vi "CombiningVIs.vi"() -> ()   [LabVIEW 2012]
uses:
  SubVIs/LVPresent_Globals.vi
  BotSpeakSubs/BotspeakSettingsUsed.vi
panel:
  in  "State 2":enum16{"LO", "HI"}(ring)=enum."HI"
  in  "Open":bool
  in  "Port":u8=13
  in  "State":enum16{"LO", "HI"}(ring)
  in  "Run":bool
  # "Combining VIs\n\nYou can add multiple VIs together on the diagram - and if you wire them together, the pink line defines the order in which things execute.  Wires contain data, and the second VI on a string cannot run until the first is complete and puts data on the pink wire.  If there were no wire, both VIs would run at the same time.  First click the Run button again, and then try opening the VI and playing around with the code."
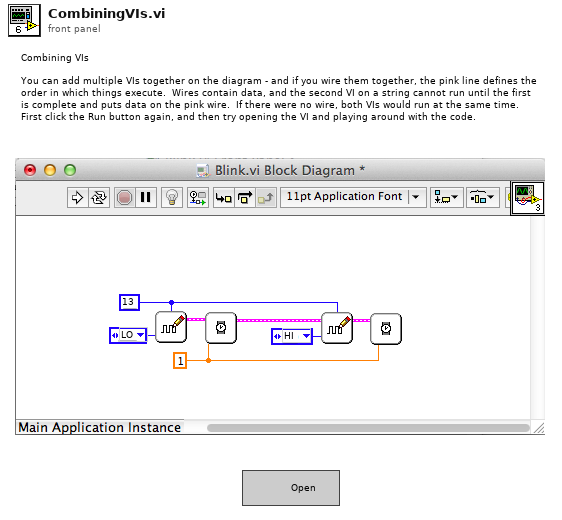
[diagram p1: front panel]
types:
  T1 = typedef "BotSpeak_Control.ctl" = cluster{"Address":string, "Reply EOF":string, "Hardware":string, "Retries":i8, "Timeout":i32, "Open?":bool}
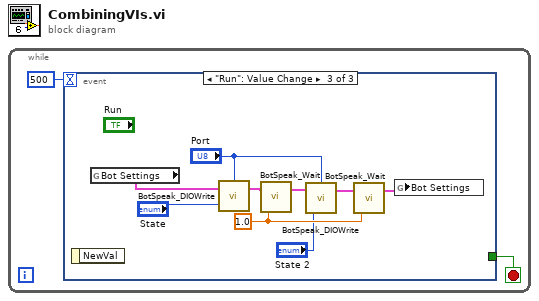
[diagram p0: block diagram]
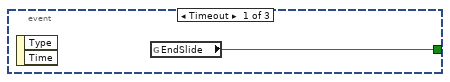
[diagram p2: hidden frame]
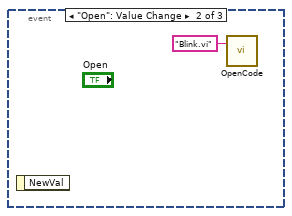
[diagram p3: hidden frame]
diagram:
  n1 = while {
    stop <- w2 stop-if-true
    n2 = event shown="[2] \"Run\": Value Change" {
      selector: _ -> [_ _ _]
      dyn-events: _ -> [_ _ _]
      timeout: 500 -> [_ _ _]
      tunnel: [w3 _ _] -> w2
      event Timeout {
        n3 = event-data() -> ()  [unwired: 1 in, 2 out]
        n4 = global read "LVPresent_Globals.vi" "EndSlide"() -> (w3:bool)
      }
      event "Open": Value Change {
        n5 = event-data() -> ()  [unwired: 1 in, 1 out]
        n6 = call "OpenCode.vi"("Code name"="Blink.vi") -> ()  [unwired: 3 in]
      }
      event "Run": Value Change {
        w9 = 1.0 ("Wait (sec)")
        n7 = event-data() -> ()  [unwired: 1 in, 1 out]
        n8 = global read "BotspeakSettingsUsed.vi" "Bot Settings"() -> (w6:T1)
        n9 = call <userlib>:"BotSpeak_DIOWrite.vi"("State"="State", "Bot Settings"=w6, "DIO Line"="Port") -> ("Bot Settings"=w12:T1)  [unwired: 1 out]
        n10 = call <userlib>:"BotSpeak_Wait.vi"("Wait (sec)"=w9, "Bot Settings"=w12) -> ("Bot Settings"=w11:T1)  [unwired: 1 in]
        n11 = call <userlib>:"BotSpeak_DIOWrite.vi"("State"="State 2", "Bot Settings"=w11, "DIO Line"="Port") -> ("Bot Settings"=w10:T1)  [unwired: 1 out]
        n12 = call <userlib>:"BotSpeak_Wait.vi"("Wait (sec)"=w9, "Bot Settings"=w10) -> ("Bot Settings"=w5:T1)  [unwired: 1 in]
        n13 = global write "BotspeakSettingsUsed.vi" "Bot Settings"(w5) -> ()
      }
    }
  }
